vi "Initialize.vi"(8 "error in (no error)":errorcluster, 11 "RP Lockin in":refnum<class "RP Transceiver.lvclass">) -> (0 "error out":errorcluster, 3 "RP Lockin out":refnum<class "RP Transceiver.lvclass">)   [LabVIEW 2015, in "RP Transceiver.lvclass"]
uses:
  RP Transceiver.lvclass
  RP Command.ctl
  RP Transceiver.lvclass/RP Transceiver.ctl
  RP Communicator/RP Communicator.lvclass
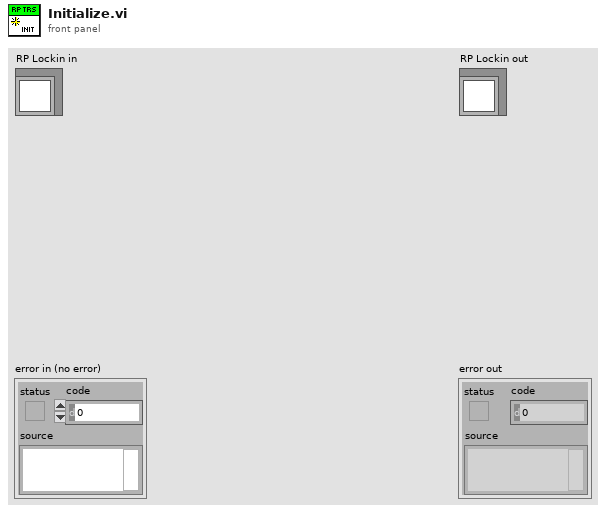
[diagram p1: front panel]
types:
  T1 = typedef "RP Command.ctl" = enum16{"Set frequency", "Read IDN", "Stop server", "Get status", "Get temperature", "Connect client", "Arm", "Software trigger", "Get whole buffer", "Get chunk", "System call", "Get config", "Set config", "Recieve data", "Play pattern", "Transmit data"}
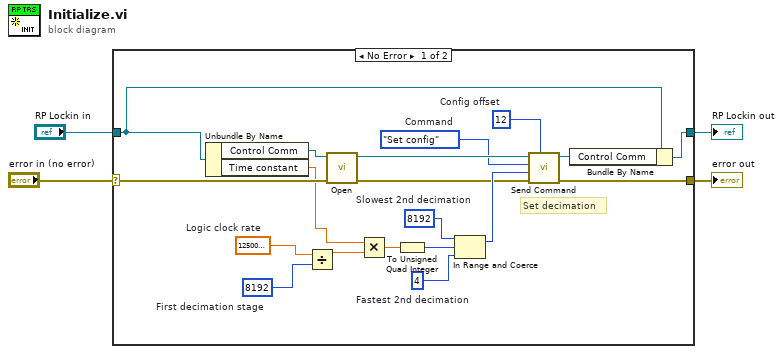
[diagram p0: block diagram]
diagram:
  n1 = case shown="No Error" "error in (no error)" {
    selector: "error in (no error)" -> [w21 w25]
    tunnel: [w6 w25] -> w3
    tunnel: [w20 w24] -> w1
    tunnel: "RP Lockin in" -> [w23 w24]
    frame No Error {
      w5 = u64 8192  # Slowest 2nd decimation
      w8 = u64 12  # Config offset
      w9 = RP_Command."Set config"  # Command
      w12 = u64 8192  # First decimation stage
      w11 = u64 4  # Fastest 2nd decimation
      w17 = 125000000.0  # Logic clock rate
      # "Set decimation"
      n2 = Unbundle By Name(w23) -> ("Control Comm"=w22:refnum<class "RP Communicator.lvclass">, "Time constant"=w15:dbl)
      n3 = Divide(x=w17, y=w12) -> (x/y=w16:dbl)
      n4 = call-dynamic "Open.vi"("error in (no error)"=w21, "RP Communicator in"=w22) -> ("error out"=w7:errorcluster, "RP Communicator out"=w19:refnum<class "RP Communicator.lvclass">)  [unwired: 8 in]
      n5 = Multiply(x=w15, y=w16) -> (x*y=w14:dbl)
      n6 = To Unsigned Quad Integer(1:w14) -> (0:w13:u64)
      n7 = In Range and Coerce(upper limit=w5, x=w13, lower limit=w11) -> (coerced(x)=w10:u64)  [unwired: 1 out]
      n8 = call-dynamic "Send Command.vi"("Config offset"=w8, "error in (no error)"=w7, "Command payload"=w10, "Command number"=w9, "RP Communicator in"=w19) -> ("error out"=w6:errorcluster, "RP Communicator out"=w18:refnum<class "RP Communicator.lvclass">)  [unwired: 5 in]
      n9 = Bundle By Name(cluster=w23, "Control Comm"=w18) -> (w20:refnum<class "RP Transceiver.lvclass">)
    }
    frame Error {
    }
  }
  "error out" <- w3
  "RP Lockin out" <- w1
